vi "Phasor Rotation due to Offset.vi"(6 "t0":ext, 9 "dt":ext, 10 "T":ext, 11 "j 2 pi f":cxt) -> (3 "exp(i 2 pi f theta_0)":cxt)   [LabVIEW 2019]
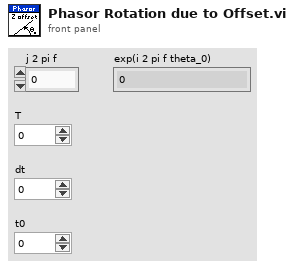
[diagram p1: front panel]
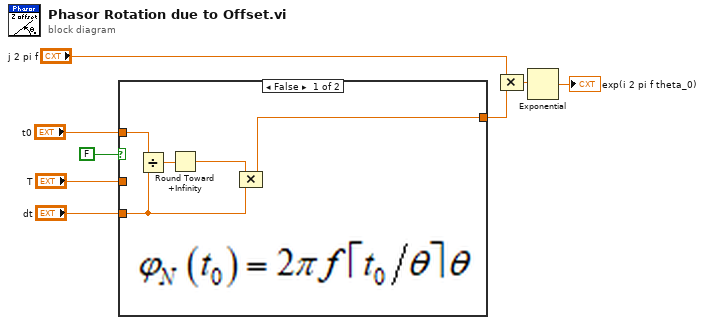
[diagram p0: block diagram]
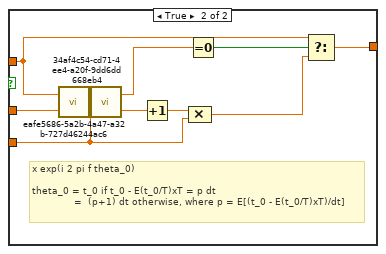
[diagram p2: hidden frame]
diagram:
  n1 = case shown="False" FALSE {
    tunnel: "dt" -> [w10 w23]
    tunnel: [w9 w19] -> w3
    tunnel: "t0" -> [w13 w17]
    tunnel: "T" -> [_ w14]
    frame False {
      n2 = Divide(x=w13, y=w10) -> (x/y=w12:ext)
      n3 = Round Toward +Infinity(x=w12) -> (ceil(x): smallest int >= x=w11:ext)
      n4 = Compound Arithmetic op=MULTIPLY(w11, w10) -> (w9:ext)
    }
    frame True {
      # "x exp(i 2 pi f theta_0)\n\ntheta_0 = t_0 if t_0 - E(t_0/T)xT = p dt\n              =  (p+1) dt otherwise, where p = E[(t_0 - E(t_0/T)xT)/dt]"
      n5 = call "eafe5686-5a2b-4a47-a32b-727d46244ac6.vi"("y"=w14, "x"=w17) -> ("x - E(x/y)y"=w15:ext)  [unwired: 1 out]
      n6 = call "34af4c54-cd71-4ee4-a20f-9dd6dd668eb4.vi"("y"=w23, "x"=w15) -> ("E(x/y)"=w20:ext, "x - E(x/y)y"=w16:ext)
      n7 = Increment(x=w20) -> (x+1=w21:ext)
      n8 = Equal To 0?(x=w16) -> (x = 0?=w18:bool)
      n9 = Compound Arithmetic op=MULTIPLY(w21, w23) -> (w22:ext)
      n10 = Select(t=w17, s=w18, f=w22) -> (s? t:f=w19:ext)
    }
  }
  n11 = Compound Arithmetic op=MULTIPLY("j 2 pi f", w3) -> (w2:cxt)
  n12 = Exponential(1:w2) -> (0:→"exp(i 2 pi f theta_0)":cxt)
